vi "motion test.vi"() -> ()   [LabVIEW 2020]
uses:
  Classes/Controller/Controller.lvclass
  Classes/Controller/Motion/Motion.lvclass
panel:
  out "error out":errorcluster
  in  "error in (no error)":errorcluster
  in  "stop":bool
  in  "XYZTheta In":dbl[](array[numeric])
  in  "Go":bool
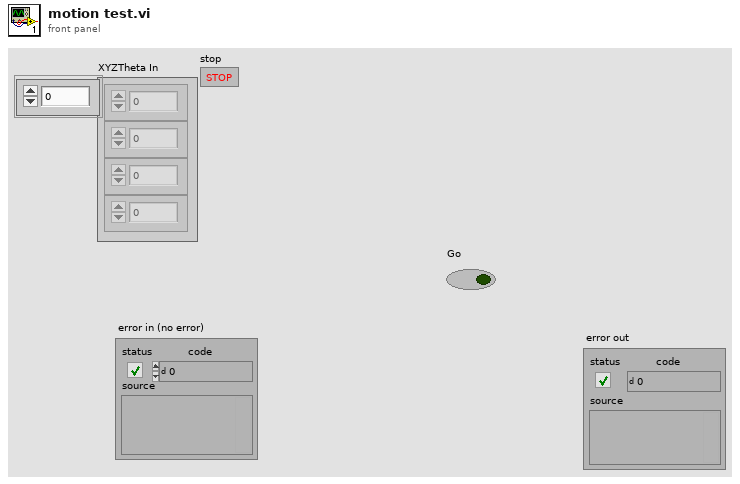
[diagram p1: front panel]
types:
  T1 = typedef "Controller.lvclass/Controllers.ctl" = cluster{"I-O.lvclass":refnum<class "I-O.lvclass">, "Gantry":refnum<k24>, "Dispenser":refnum<visa-resource-name>}
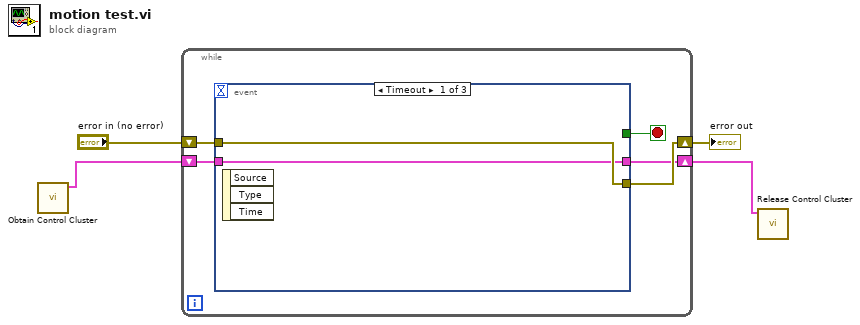
[diagram p0: block diagram]
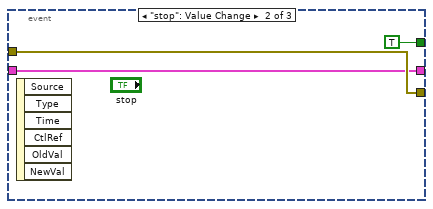
[diagram p2: hidden frame]
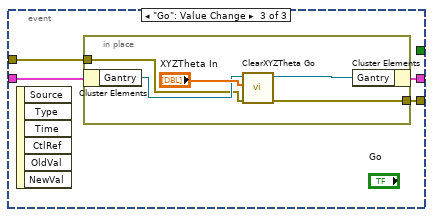
[diagram p3: hidden frame]
diagram:
  n1 = call "Obtain Control Cluster.vi"() -> ("Control Out"=w4:T1)  [unwired: 11 in]
  n2 = while {
    shift-right: [w6] -> w2
    shift-left: "error in (no error)" -> [w7]
    shift-right: [w5] -> w1
    shift-left: w4 -> [w9]
    stop <- w8 stop-if-true
    n3 = event shown="[0] Timeout" {
      selector: _ -> [_ _ _]
      dyn-events: _ -> [_ _ _]
      timeout: _ -> [_ _ _]
      tunnel: w9 -> [w10 w12 w18]
      tunnel: [_ TRUE _] -> w8
      tunnel: w7 -> [w11 w13 w17]
      tunnel: [w11 w13 w16] -> w6
      tunnel: [w10 w12 w15] -> w5
      event Timeout {
        n4 = event-data() -> ()  [unwired: 1 in, 3 out]
      }
      event "stop": Value Change {
        n5 = event-data() -> ()  [unwired: 1 in, 6 out]
      }
      event "Go": Value Change {
        n6 = event-data() -> ()  [unwired: 1 in, 6 out]
        n7 = in-place {
          in-place-border: w17 -> [w20]
          in-place-border: [w19] -> w16
          n8 = in-place-cluster #1(w18) -> ("Gantry"=w21:refnum<k24>)
          n9 = call "ClearXYZTheta Go.vi"("error in (no error)"=w20, "XYZTheta In"="XYZTheta In", "Gantry In"=w21) -> ("error out"=w19:errorcluster, "Gantry Out"=w22:refnum<k24>)  [unwired: 6 in, 1 out]
          n10 = in-place-cluster #1("Gantry"=w22) -> (w15:T1)
        }
      }
    }
  }
  "error out" <- w2
  n11 = call "Release Control Cluster.vi"("output cluster"=w1) -> ()  [unwired: 11 in]
